vi "SM Init.vi"(9 "Status In":T1={"State"=enum."Idle", "Motor"={"#1"=FALSE, "#2"=FALSE, "#3"=FALSE}, "Timer"=30.0}) -> (0 "State":T2, 1 "Status Out":T1={"State"=enum."Idle", "Motor"={"#1"=FALSE, "#2"=FALSE, "#3"=FALSE}, "Timer"=30.0}, 3 "State Changed":bool caption="已更改")   [LabVIEW 2013]
uses:
  Control/Data.ctl
  Control/State.ctl
  Control/Motor.ctl
  <vilib>/ptbypt/NI_PtbyPt.lvlib
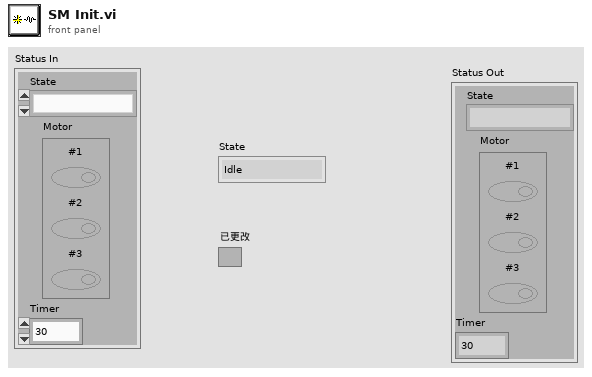
[diagram p1: front panel]
types:
  T1 = typedef "Data.ctl" = cluster{"State":T2, "Motor":T3, "Timer":dbl}
  T2 = typedef "State.ctl" = enum16{"Idle", "#1 Run", "#2 Run", "#3 Run", "#3 Stop", "#2 Stop", "#1 Stop"}
  T3 = typedef "Motor.ctl" = cluster{"#1":bool, "#2":bool, "#3":bool}
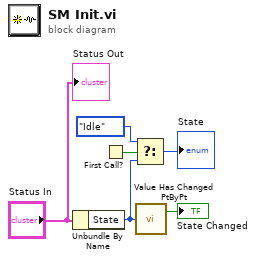
[diagram p0: block diagram]
diagram:
  n1 = Unbundle By Name("Status In") -> ("State"=w2:T2)
  n2 = First Call?() -> (First Call?: T/F=w4:bool)
  n3 = Select(t=State."Idle" ("State"), s=w4, f=w2) -> (s? t:f=→"State":T2)
  n4 = call <vilib>:"Value Has Changed PtByPt.vi"("input data point"=w2) -> ("has changed"=→"State Changed":bool)  [unwired: 1 in, 1 out]
  "Status Out" <- "Status In"
